vi "FindElementStartByName_NIMOD.vi"(6 "offset (0)":i32, 8 "max offset":i32, 9 "ignore empty elements? (false)":bool, 10 "Element Name":string, 11 "string":string) -> (4 "offset past match":i32)   [LabVIEW 2011]
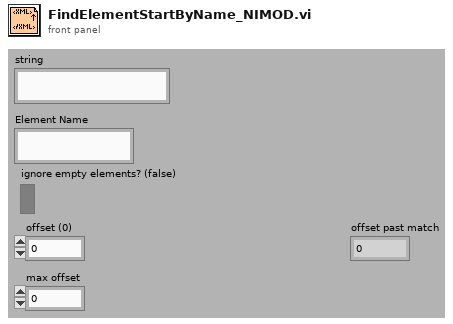
[diagram p1: front panel]
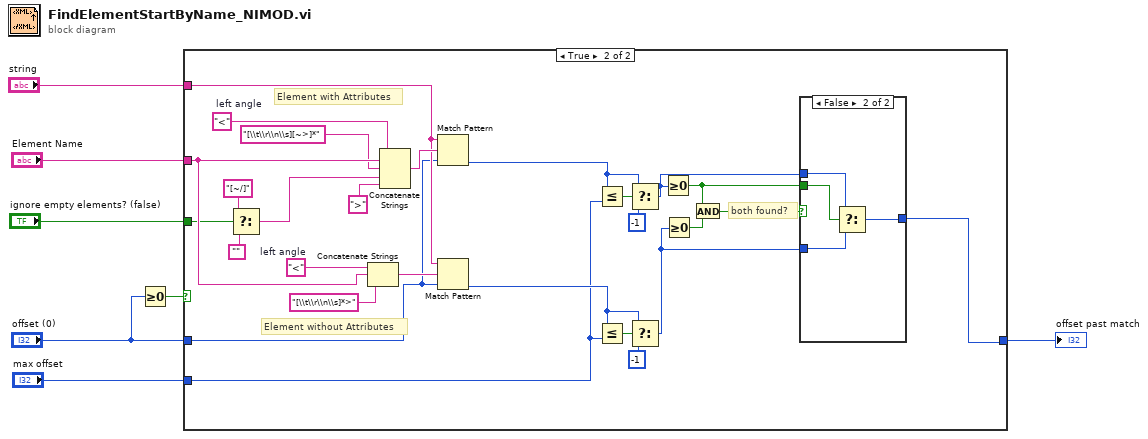
[diagram p0: block diagram]
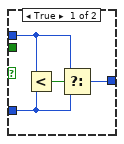
[diagram p3: hidden frame]
diagram:
  n1 = Greater Or Equal To 0?(x="offset (0)") -> (x >= 0?=w1:bool)
  n2 = case shown="True" w1 {
    tunnel: [w8 w16] -> w7
    tunnel: "Element Name" -> [_ w32]
    tunnel: "ignore empty elements? (false)" -> [_ w24]
    tunnel: "max offset" -> [_ w18]
    tunnel: "string" -> [_ w14]
    tunnel: "offset (0)" -> [w8 w12]
    frame False {
    }
    frame True {
      w33 = "<"  # left angle
      w35 = "<"  # left angle
      # "Element without Attributes"
      # "Element with Attributes"
      # "both found?"
      n3 = Select(t="[~/]" ("regular expression"), s=w24, f="") -> (s? t:f=w10:string)
      n4 = Concatenate Strings(w33, w32, "[\\t\\r\\n\\s]*>" ("regular expression")) -> (w30:string)
      n5 = Concatenate Strings(w35, w32, "[\\t\\r\\n\\s][~>]*" ("regular expression"), w10, ">" ("regular expression")) -> (w34:string)
      n6 = Match Pattern(string=w14, regular expression=w34, offset (0)=w12) -> (offset past match=w13:i32)  [unwired: 3 out]
      n7 = Match Pattern(string=w14, regular expression=w30, offset (0)=w12) -> (offset past match=w22:i32)  [unwired: 3 out]
      n8 = Less Or Equal?(x=w13, y=w18) -> (x <= y?=w19:bool)
      n9 = Less Or Equal?(x=w22, y=w18) -> (x <= y?=w23:bool)
      n10 = Select(t=w13, s=w19, f=-1) -> (s? t:f=w17:i32)
      n11 = Select(t=w22, s=w23, f=-1) -> (s? t:f=w15:i32)
      n12 = Greater Or Equal To 0?(x=w17) -> (x >= 0?=w27:bool)
      n13 = Greater Or Equal To 0?(x=w15) -> (x >= 0?=w29:bool)
      n14 = And(x=w27, y=w29) -> (x .and. y?=w28:bool)
      n15 = case shown="False" w28 {
        tunnel: w17 -> [w38 w40]
        tunnel: w15 -> [w36 w41]
        tunnel: w27 -> [_ w42]
        tunnel: [w39 w43] -> w16
        frame True {
          n16 = Less?(x=w38, y=w36) -> (x < y?=w37:bool)
          n17 = Select(t=w38, s=w37, f=w36) -> (s? t:f=w39:i32)
        }
        frame False {
          n18 = Select(t=w40, s=w42, f=w41) -> (s? t:f=w43:i32)
        }
      }
    }
  }
  "offset past match" <- w7
